vi "Pre-Install Custom Action.vi"(10 "Variant":variant) -> (0 "error out":errorcluster)   [LabVIEW 2014]
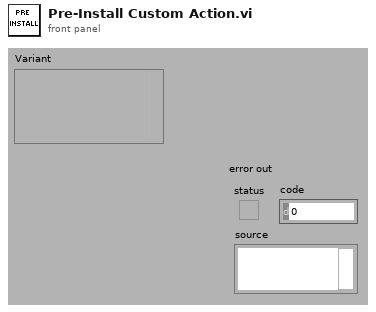
[diagram p1: front panel]
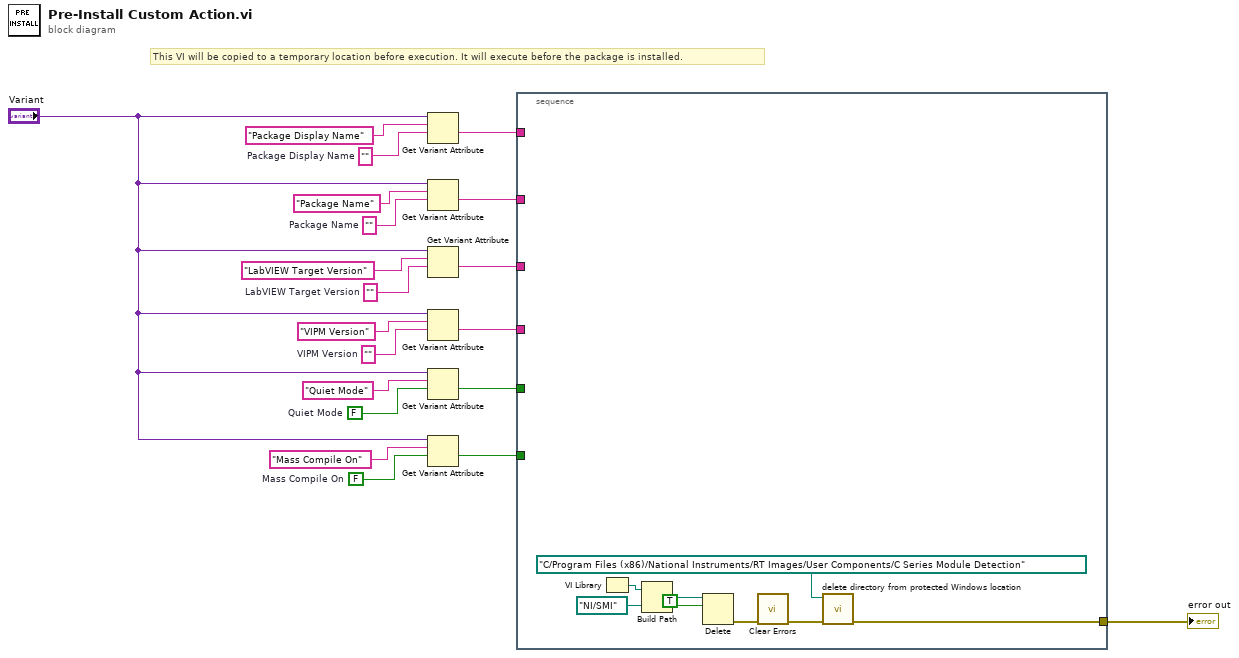
[diagram p0: block diagram]
diagram:
  w2 = FALSE  # Mass Compile On
  w4 = ""  # Package Display Name
  w11 = FALSE  # Quiet Mode
  w14 = ""  # VIPM Version
  w16 = ""  # LabVIEW Target Version
  w18 = ""  # Package Name
  # "This VI will be copied to a temporary location before execution. It will execute before the package is installed."
  n1 = Get Variant Attribute(Variant="Variant", name="Package Display Name", default value (empty Variant)=w4) -> (value=w10:string)  [unwired: 1 in, 3 out]
  n2 = Get Variant Attribute(Variant="Variant", name="Package Name", default value (empty Variant)=w18) -> (value=w9:string)  [unwired: 1 in, 3 out]
  n3 = Get Variant Attribute(Variant="Variant", name="LabVIEW Target Version", default value (empty Variant)=w16) -> (value=w8:string)  [unwired: 1 in, 3 out]
  n4 = Get Variant Attribute(Variant="Variant", name="VIPM Version", default value (empty Variant)=w14) -> (value=w7:string)  [unwired: 1 in, 3 out]
  n5 = Get Variant Attribute(Variant="Variant", name="Quiet Mode", default value (empty Variant)=w11) -> (value=w6:bool)  [unwired: 1 in, 3 out]
  n6 = Get Variant Attribute(Variant="Variant", name="Mass Compile On", default value (empty Variant)=w2) -> (value=w5:bool)  [unwired: 1 in, 3 out]
  n7 = stacked-sequence {
    tunnel: w10 -> [_]
    tunnel: w9 -> [_]
    tunnel: w8 -> [_]
    tunnel: w7 -> [_]
    tunnel: w6 -> [_]
    tunnel: w5 -> [_]
    tunnel: [w21] -> w1
    frame #0 {
      n8 = VI Library() -> (path=w27:path)
      n9 = Build Path(base path=w27, name or relative path=path "NI/SMI") -> (appended path=w25:path)
      n10 = Delete(path (use dialog)=w25, entire hierarchy (F)=TRUE) -> (error out=w23:errorcluster)  [unwired: 3 in, 2 out]
      n11 = call <vilib>:"Clear Errors.vi"("error in (no error)"=w23) -> ("error out"=w22:errorcluster)  [unwired: 5 in, 1 out]
      n12 = call "delete directory from protected Windows location.vi"("error in"=w22, "directory"=path "C:/Program Files (x86)/National Instruments/RT Images/User Components/C Series Module Detection") -> ("error out"=w21:errorcluster)  [unwired: 8 in, 1 out]
    }
  }
  "error out" <- w1
